vi "Get API.vi"(8 "error in (no error)":errorcluster, 11 "Template Artifex in":refnum<class "Template.lvclass">) -> (0 "error out":errorcluster, 2 "Actor API":refnum<class "Actor API.lvclass">, 3 "Template Artifex out":refnum<class "Template.lvclass">)   [LabVIEW 2022 SP3, in "Artifex Template.lvlib" / "Template.lvclass"]
uses:
  Template.lvclass
  Artifex/Actor Proxy/Actor API.lvclass
  Template.lvclass/Template.ctl
  Template API/Template API.lvclass
  C:/dev/lv/2022/lv-artifex/Artifex/Actor Proxy/Actor API.lvclass
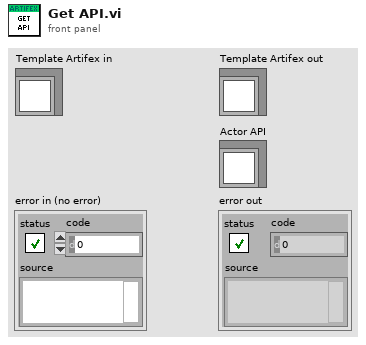
[diagram p1: front panel]
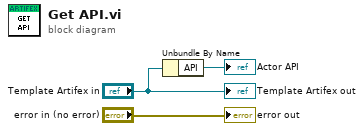
[diagram p0: block diagram]
diagram:
  n1 = Unbundle By Name("Template Artifex in") -> ("API"=→"Actor API":refnum<class "Template API.lvclass">)
  "error out" <- "error in (no error)"
  "Template Artifex out" <- "Template Artifex in"
